vi "Get Library Info.vi"(0 "reference in":refnum<class "Simulated-PowerModule.lvclass">=refnum, 11 "Error In":errorcluster) -> (4 "reference out":refnum<class "Simulated-PowerModule.lvclass">, 6 "PPL Filename":string, 8 "Build Version":string="v1.0.0.12", 15 "Error Out":errorcluster)   [LabVIEW 2023, in "Simulated-PowerModule.lvlib" / "Simulated-PowerModule.lvclass"]
uses:
  Simulated-PowerModule.lvclass
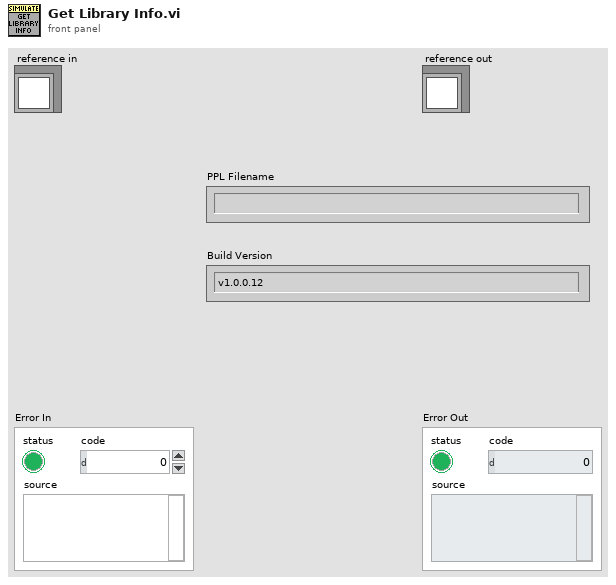
[diagram p1: front panel]
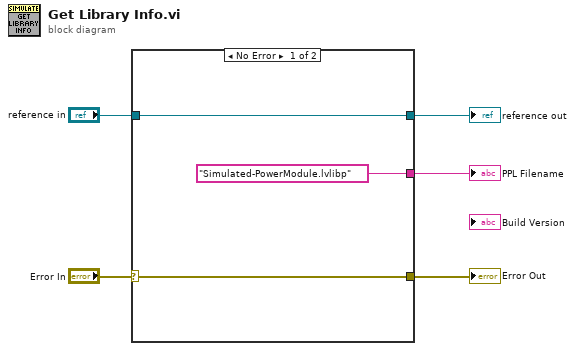
[diagram p0: block diagram]
diagram:
  n1 = case shown="No Error" "Error In" {
    selector: "Error In" -> [w6 w9]
    tunnel: ["Simulated-PowerModule.lvlibp" _] -> w5
    tunnel: [w6 w9] -> w4
    tunnel: [w8 w10] -> w3
    tunnel: "reference in" -> [w8 w10]
    frame No Error {
    }
    frame Error {
    }
  }
  "Error Out" <- w4
  "reference out" <- w3
  "PPL Filename" <- w5
